vi "Stop CMD.vi"(8 "error in (no error)":errorcluster, 10 "Message In":refnum<class "Message.lvclass">, 11 "Node Actor in":refnum<class "Node Actor.lvclass">) -> (0 "error out":errorcluster, 3 "Node Actor out":refnum<class "Node Actor.lvclass">)   [LabVIEW 2024, in "Node Actor.lvclass"]
uses:
  Node Actor.lvclass
  Node Actor.lvclass/Node Actor.ctl
  Root Actor/Root Actor.lvclass
  Message/Message.lvclass
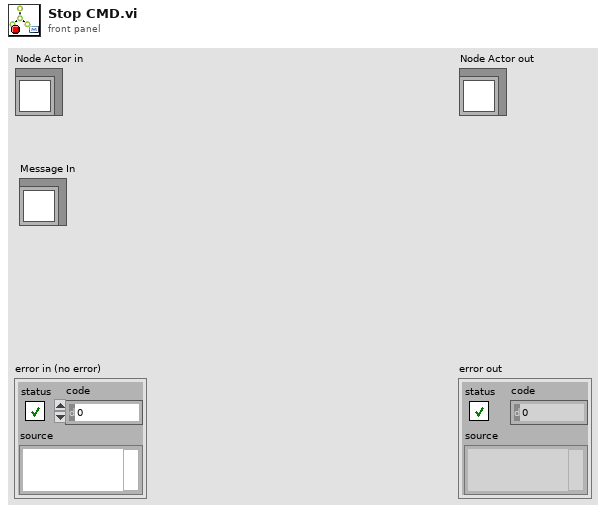
[diagram p1: front panel]
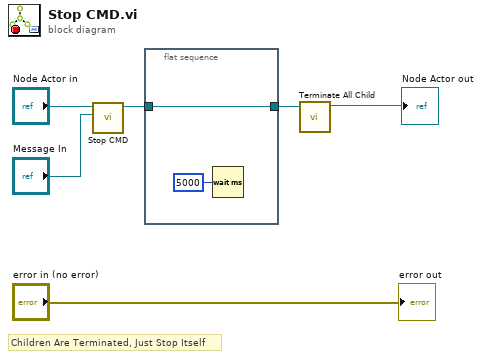
[diagram p0: block diagram]
diagram:
  # "Children Are Terminated, Just Stop Itself"
  n1 = call-parent "Stop CMD.vi"("Message In"="Message In", "Root Actor in"="Node Actor in") -> ("Root Actor out"=w3:refnum<class "Node Actor.lvclass">)  [unwired: 8 in, 1 out]
  n2 = flat-sequence {
    tunnel: w3 -> [w7]
    tunnel: [w7] -> w2
    frame #0 {
      n3 = Wait (ms)(milliseconds to wait=u32 5000) -> ()  [unwired: 1 out]
    }
  }
  n4 = call "Terminate All Child.vi"("Node Actor in"=w2) -> ("Node Actor out"=→"Node Actor out":refnum<class "Node Actor.lvclass">)  [unwired: 9 in, 1 out]
  "error out" <- "error in (no error)"
